vi "ReadFileContent.vi"(0 "VISA Refnum in":refnum<visa-resource-name>="COM1", 1 "delay Data List":u32=500, 3 "File name string 2":string="*IDN?\n", 5 "Command String":string="*IDN?\n", 7 "reference":refnum<vi>, 9 "File name string":string="*IDN?\n", 11 "delay Input":u32=500, 12 "delay Command":u32=500, 14 "delay R":u32=500) -> (4 "Array":string[](array[string]), 15 "Wrong":string[](array[string]))   [LabVIEW 2012]
uses:
  <vilib>/Instr/_visa.llb/VISA Configure Serial Port (Instr).vi
panel:
  out "x > y?":bool
  out "offset of match":i32
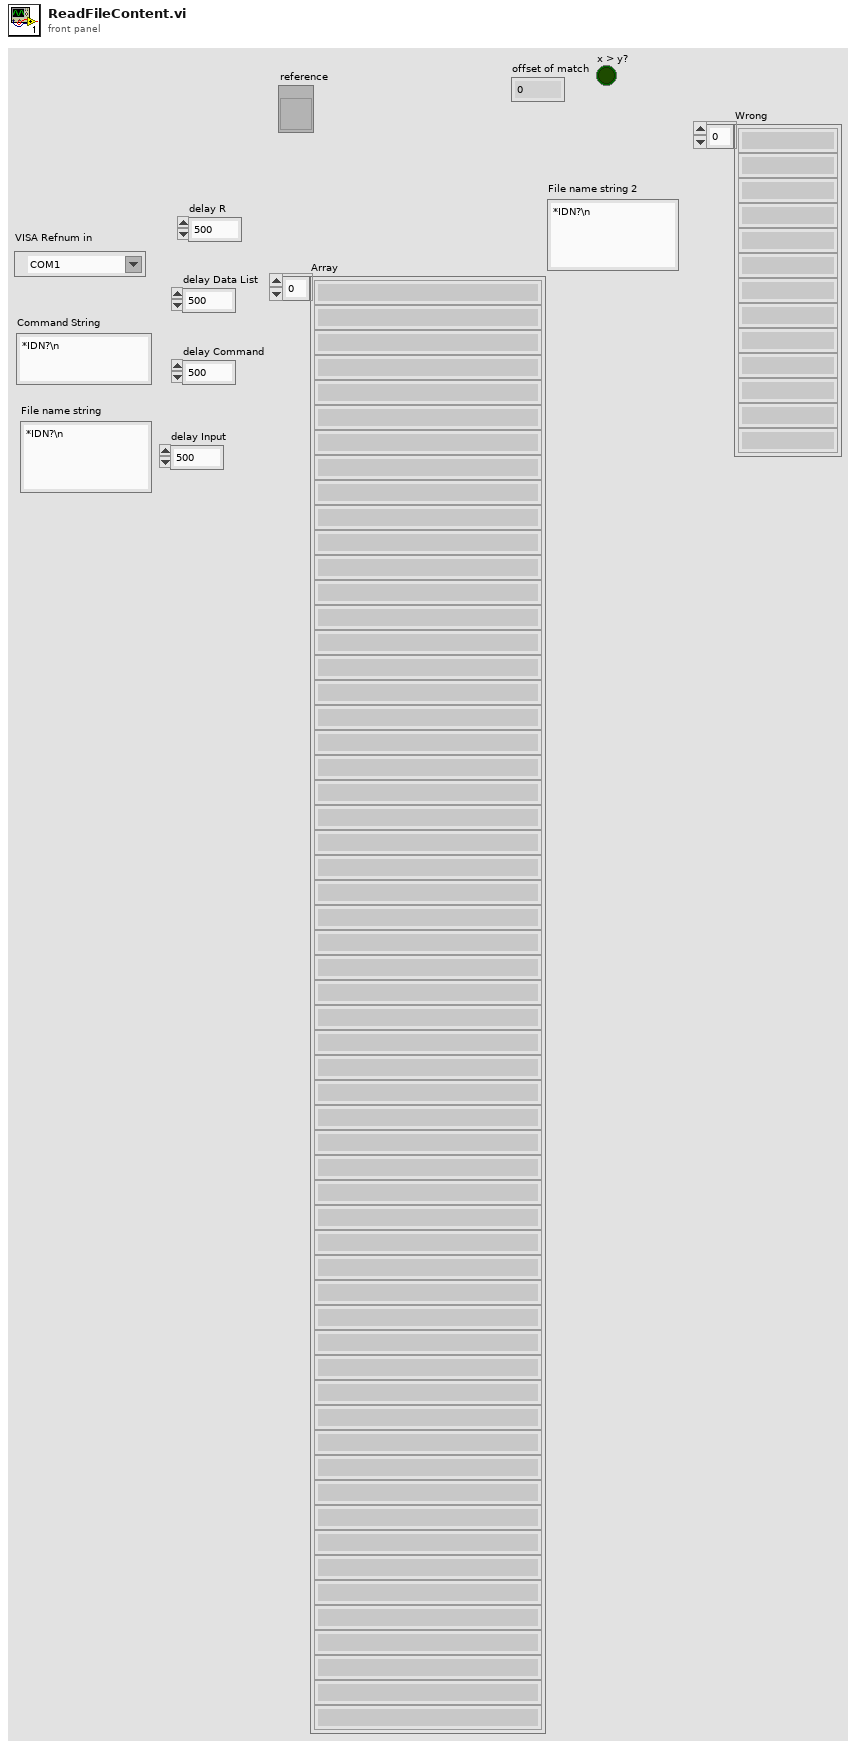
[diagram p1: front panel]
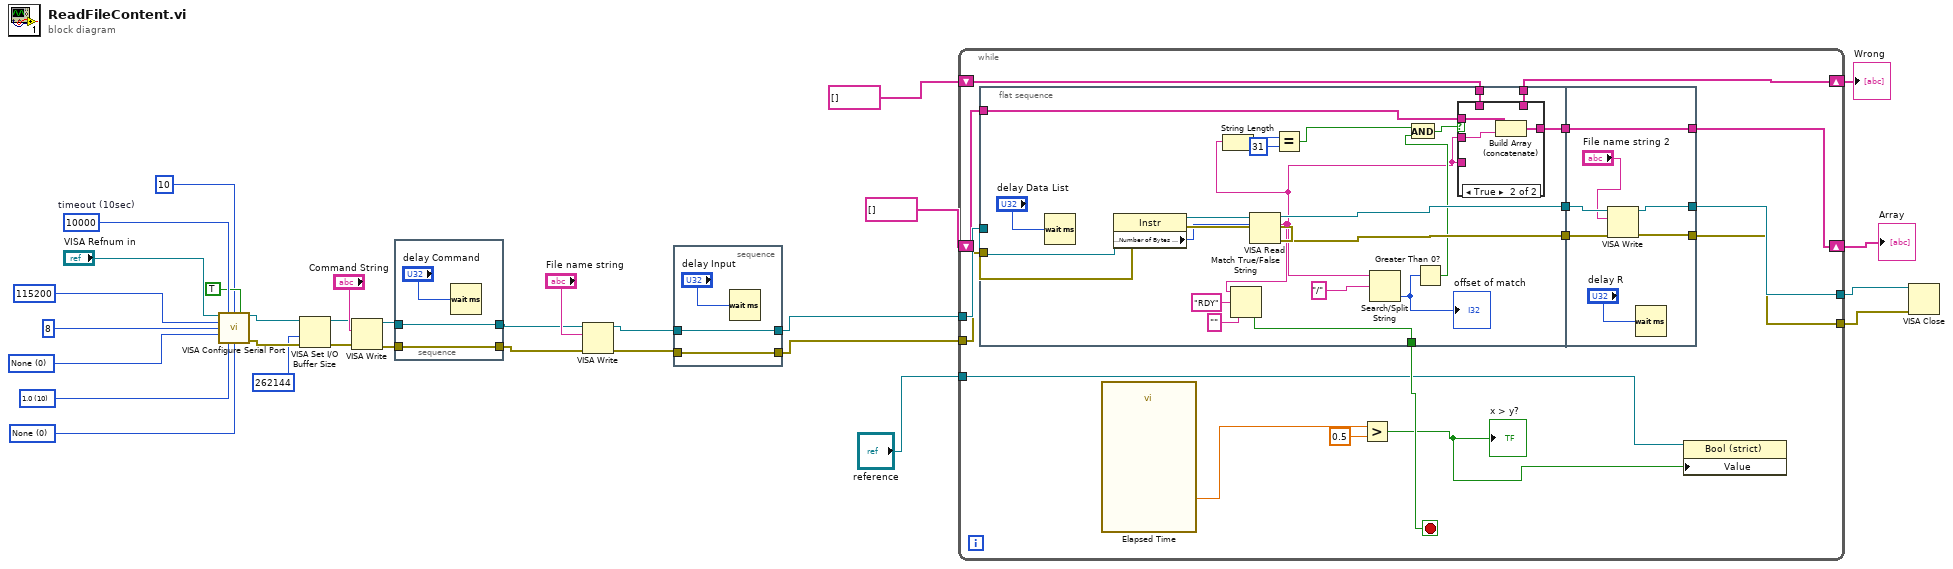
[diagram p0: block diagram]
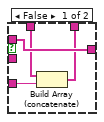
[diagram p2: hidden frame]
diagram:
  w31 = u16 0 items=["None"=0, "XON/XOFF"=1, "RTS/CTS"=2, "DTR/DSR"=4] ("flow control")
  w30 = u16 10 items=["1.0"=10, "1.5"=15, "2.0"=20] ("stop bits")
  w29 = u16 0 items=["None", "Odd", "Even", "Mark", "Space"] ("parity")
  w25 = u32 10000  # timeout (10sec)
  n1 = call-poly "VISA Configure Serial Port"("VISA resource name"="VISA Refnum in", "timeout (10sec)"=w25, "termination char\n(0xA = '\\n' = LF)"=u8 10 ("termination char\n(0xA = '\\n' = LF)"), "Enable Termination\nChar (T)"=TRUE ("Enable Termination\nChar (T)"), "baud rate (9600)"=u32 115200 ("baud rate"), "data bits (8)"=u16 8 ("data bits"), "parity (0:none)"=w29, "stop bits (10: 1 bit)"=w30, "flow control (0:none)"=w31) -> ("VISA resource name out"=w4:refnum<visa-resource-name>, "error out"=w3:errorcluster)  [unwired: 1 in, 4 out]
  n2 = VISA Set I/O Buffer Size(VISA resource name=w4, size (4096)=u32 262144, error in (no error)=w3) -> (VISA resource name out=w6:refnum<visa-resource-name>, error out=w5:errorcluster)  [unwired: 1 in]
  n3 = VISA Write(VISA resource name=w6, write buffer="Command String", error in (no error)=w5) -> (VISA resource name out=w11:refnum<visa-resource-name>, error out=w10:errorcluster)  [unwired: 1 out]
  n4 = stacked-sequence {
    tunnel: w10 -> [w34]
    tunnel: [w34] -> w16
    tunnel: w11 -> [w33]
    tunnel: [w33] -> w17
    frame #0 {
      n5 = Wait (ms)(milliseconds to wait="delay Command") -> ()  [unwired: 1 out]
    }
  }
  n6 = VISA Write(VISA resource name=w17, write buffer="File name string", error in (no error)=w16) -> (VISA resource name out=w15:refnum<visa-resource-name>, error out=w14:errorcluster)  [unwired: 1 out]
  n7 = stacked-sequence {
    tunnel: w14 -> [w37]
    tunnel: [w37] -> w12
    tunnel: w15 -> [w36]
    tunnel: [w36] -> w13
    frame #0 {
      n8 = Wait (ms)(milliseconds to wait="delay Input") -> ()  [unwired: 1 out]
    }
  }
  n9 = while {
    tunnel: [w53] -> w9
    tunnel: [w52] -> w21
    tunnel: w13 -> [w50]
    tunnel: w12 -> [w49]
    shift-right: [w44] -> w19
    shift-left: string[] [] -> [w48]
    shift-right: [w43] -> w8
    shift-left: string[] [] -> [w42]
    tunnel: "reference" -> [w39]
    stop <- w51 stop-if-true
    n10 = flat-sequence {
      tunnel: [w70] -> w51
      tunnel: w50 -> [w68]
      tunnel: w49 -> [w67]
      tunnel: w48 -> [w65]
      tunnel: [w73] -> w47
      tunnel: [w72] -> w46
      tunnel: [w66] -> w45
      tunnel: [w54] -> w43
      tunnel: w42 -> [w56]
      tunnel: [w90] -> w44
      tunnel: [w87] -> w52
      tunnel: [w86] -> w53
      tunnel: w47 -> [w89]
      tunnel: w46 -> [w88]
      tunnel: w45 -> [w90]
      frame #0 {
        n11 = Wait (ms)(milliseconds to wait="delay Data List") -> ()  [unwired: 1 out]
        n12 = property class="Instr"(reference=w68, error in=w67) -> (reference out=w76:refnum<visa-resource-name>, error out=w75:errorcluster, "Serial Settings:Number of Bytes at Serial Port"=w74:u32)
        n13 = VISA Read(VISA resource name=w76, byte count=w74, error in (no error)=w75) -> (VISA resource name out=w73:refnum<visa-resource-name>, read buffer=w55:string, error out=w72:errorcluster)  [unwired: 1 out]
        n14 = String Length(string=w55) -> (length=w60:i32)
        n15 = Match True/False String(2:"" ("false string"), 3:"RDY" ("true string"), 4:w55) -> (0:w70:bool)  [unwired: 1 out]
        n16 = Equal?(x=w60, y=31) -> (x = y?=w58:bool)
        n17 = Search/Split String(string=w55, search string/char (-)="/") -> (offset of match=w63:i32)  [unwired: 1 in, 2 out]
        "offset of match" <- w63
        n18 = Greater Than 0?(x=w63) -> (x > 0?=w61:bool)
        n19 = And(x=w58, y=w61) -> (x .and. y?=w57:bool)
        n20 = case shown="True" w57 {
          tunnel: [w80 w83] -> w66
          tunnel: w65 -> [w80 w82]
          tunnel: w55 -> [_ w81]
          tunnel: w56 -> [w79 _]
          tunnel: w55 -> [w78 _]
          tunnel: [w77 _] -> w54
          frame False {
            n21 = Build Array (concatenate)(w79, w78) -> (w77:string[])
          }
          frame True {
            n22 = Build Array (concatenate)(w82, w81) -> (w83:string[])
          }
        }
      }
      frame #1 {
        n23 = VISA Write(VISA resource name=w89, write buffer="File name string 2", error in (no error)=w88) -> (VISA resource name out=w86:refnum<visa-resource-name>, error out=w87:errorcluster)  [unwired: 1 out]
        n24 = Wait (ms)(milliseconds to wait="delay R") -> ()  [unwired: 1 out]
      }
    }
    n25 = call "Elapsed Time"() -> ("Elapsed Time (s)"=w40:dbl)  [unwired: 12 in, 7 out]
    n26 = Greater?(x=w40, y=0.5) -> (0:w38:bool)
    "x > y?" <- w38
    n27 = property class="Bool (strict)"(reference=w39, "Value"=w38) -> ()  [unwired: 1 in, 2 out]
  }
  "Array" <- w19
  "Wrong" <- w8
  n28 = VISA Close(VISA resource name=w9, error in (no error)=w21) -> ()  [unwired: 1 out]
